vi "AR Drone - Simple Control.vi"() -> ()   [LabVIEW 2014]
doc: "Very simple example showing how to use the base VIs to control the AR Drone."
uses:
  <vilib>/LVH/AR Drone Toolkit/AR Drone.lvlib
panel:
  out "Control Cluster":T1 {"Roll" scale=-1.0..1.0; "Pitch" scale=-1.0..1.0; "Vertical Speed" scale=-1.0..1.0; "Yaw Speed" scale=-1.0..1.0}
  in  "Setup Parameters":T2={"Drone IP address"="192.168.1.1", "Home IP address"="192.168.1.2", "Flight Mode"=enum."INDOOR MODE", "Mounted Hull"=enum."INDOOR HULL", "Video Camera"=2, "Max Altitude (m)"=3.0, "Max Pitch and Roll Angle (deg)"=10.0, "Max Vertical Speed (m/s)"=0.7, "Max Yaw Speed (deg/s)"=100.0} {"Video Camera" items=["Bottom Camera"=1, "Front Camera"=0, "Front in Bottom"=3, "Bottom in Front"=2]}
  in  "Speed step":dbl=0.5
  in  "stop":bool
  in  "Emergency Landing":bool
  in  "Take Off/Land":bool
  in  "Hover":bool
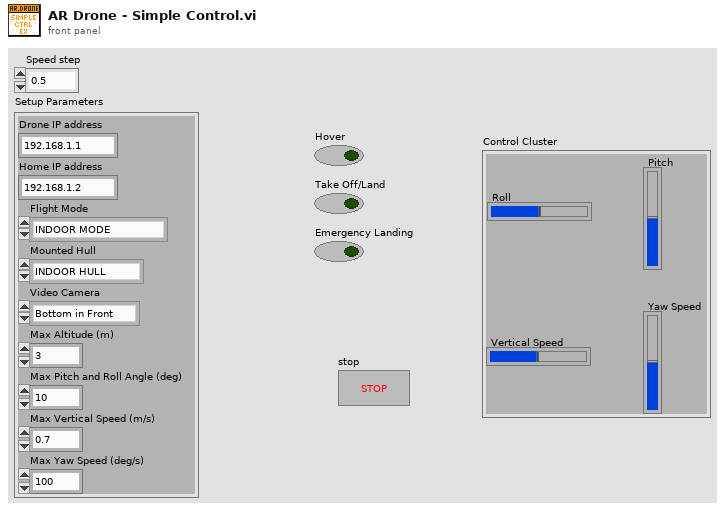
[diagram p1: front panel]
types:
  T1 = cluster{"Roll":dbl, "Pitch":dbl, "Vertical Speed":dbl, "Yaw Speed":dbl}
  T2 = cluster{"Drone IP address":string, "Home IP address":string, "Flight Mode":enum8{"OUTDOOR MODE", "INDOOR MODE"}, "Mounted Hull":enum8{"OUTDOOR HULL", "INDOOR HULL"}, "Video Camera":u8, "Max Altitude (m)":sgl, "Max Pitch and Roll Angle (deg)":sgl, "Max Vertical Speed (m/s)":sgl, "Max Yaw Speed (deg/s)":sgl}
  T3 = typedef "AR Drone.lvlib/AR Drone Resource.ctl" = cluster{"UDP Control Connection":refnum<k16>, "UDP NavData Connection":refnum<k16>, "UDP Video Connection (Drone 1.0)":refnum<k16>, "TCP Video Connection (Drone 2.0)":refnum<k5>, "TCP Control Port Connection":refnum<k5>, "Drone IP address":string, "Drone Command Port":u16, "Drone NavData Port":u16, "Drone Vid Stream Port":u16, "Drone TCP Control Port":u16, "Home IP address":string, "Home Command Port":u16, "Home NavData Port":u16, "Home Vid Stream Port":u16, "Drone Version":i32, "Drone Index":i32, "Command Sequence":i32}
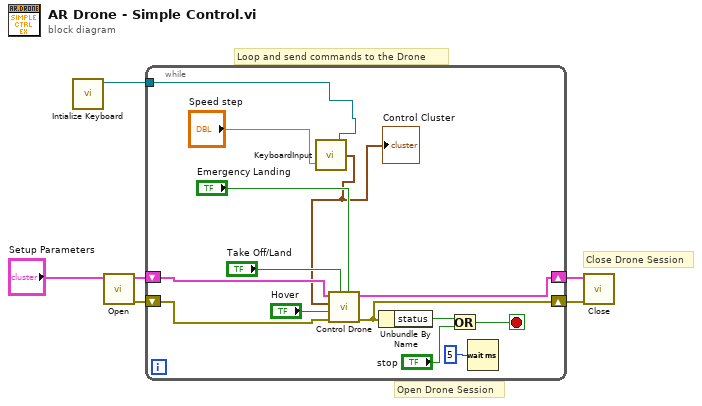
[diagram p0: block diagram]
diagram:
  # "Close Drone Session"
  # "Loop and send commands to the Drone"
  # "Open Drone Session"
  n1 = call <vilib>:"Intialize Keyboard.vi"() -> ("device ID"=w1:refnum<k1>)  [unwired: 10 in, 1 out]
  n2 = call <vilib>:"Open.vi"("Setup Parameters"="Setup Parameters") -> ("error out"=w6:errorcluster, "AR Drone Resource"=w5:T3)  [unwired: 9 in]
  n3 = while {
    shift-right: [w15] -> w4
    shift-left: w5 -> [w19]
    shift-right: [w10] -> w3
    shift-left: w6 -> [w20]
    tunnel: w1 -> [w7]
    stop <- w11 stop-if-true
    n4 = call "KeyboardInput.vi"("Speed step"="Speed step", "device ID"=w7) -> ("Control cluster"=w8:T1)  [unwired: 1 in, 1 out]
    "Control Cluster" <- w8
    n5 = call <vilib>:"Control Drone.vi"("Emergency Landing"="Emergency Landing", "Takeoff/Land"="Take Off/Land", "error in (no error)"=w20, "Hover"="Hover", "Control Cluster"=w8, "AR Drone Resource"=w19) -> ("error out"=w10:errorcluster, "AR Drone Resource Out"=w15:T3)  [unwired: 4 in]
    n6 = Unbundle By Name(w10) -> ("status"=w13:bool)
    n7 = Or(x=w13, y="stop") -> (x .or. y?=w11:bool)
    n8 = Wait (ms)(milliseconds to wait=u32 5) -> ()  [unwired: 1 out]
  }
  n9 = call <vilib>:"Close.vi"("error in (no error)"=w3, "AR Drone Resource"=w4) -> ()  [unwired: 9 in, 1 out]
